vi "ReadFile.vi"(8 "error in (no error)":errorcluster, 11 "VXMCfg in":refnum<class "VXMCfg.lvclass">) -> (0 "error out":errorcluster, 3 "VXMCfg out":refnum<class "VXMCfg.lvclass">)   [LabVIEW 2018, in "VXMCfg.lvclass"]
uses:
  VXMCfg.lvclass
  VXMCfg.ctl
  sub-syst.n.ctl
  VXMCfg.lvclass/VXMCfg.ctl
panel:
  in  "VXM Properties":T1={"sub-syst1"={"Addr"="COM11", "Enable"=TRUE, "X scale eng./step"=0.00635, "Y scale eng./step"=0.00635, "Z scale eng./step"=0.0125, "T scale eng./step"=1.0, "X units"="mm", "Y units"="mm", "Z units"="deg", "T units"="", "X Jog"=1.0, "Y Jog"=1.0, "Z Jog"=1.0, "T Jog"=1.0, "X-1 Name"="", "Y-2 Name"="", "Z-3 Name"="", "T-4 Name"="", "VXM (1-4)"=3}, "sub-syst2"={"Addr"="", "Enable"=FALSE, "X scale eng./step"=0.00635, "Y scale eng./step"=0.00635, "Z scale eng./step"=0.0125, "T scale eng./step"=0.0125, "X units"="mm", "Y units"="mm", "Z units"="deg", "T units"="deg", "X Jog"=1.0, "Y Jog"=1.0, "Z Jog"=1.0, "T Jog"=1.0, "X-1 Name"="", "Y-2 Name"="", "Z-3 Name"="", "T-4 Name"="", "VXM (1-4)"=4}, "sub-syst3"={"Addr"="", "Enable"=FALSE, "X scale eng./step"=0.00635, "Y scale eng./step"=0.0125, "Z scale eng./step"=1.0, "T scale eng./step"=1.0, "X units"="mm", "Y units"="deg", "Z units"="", "T units"="", "X Jog"=1.0, "Y Jog"=1.0, "Z Jog"=1.0, "T Jog"=1.0, "X-1 Name"="", "Y-2 Name"="", "Z-3 Name"="", "T-4 Name"="", "VXM (1-4)"=2}}
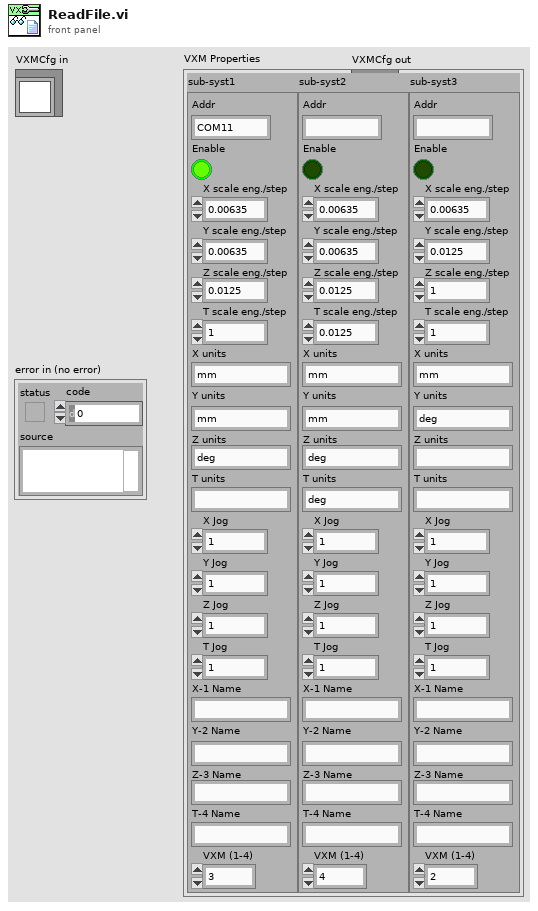
[diagram p1: front panel]
types:
  T1 = typedef "VXMCfg.ctl" = cluster{"sub-syst1":T2, "sub-syst2":T2, "sub-syst3":T2}
  T2 = typedef "sub-syst.n.ctl" = cluster{"Addr":string, "Enable":bool, "X scale eng./step":dbl, "Y scale eng./step":dbl, "Z scale eng./step":dbl, "T scale eng./step":dbl, "X units":string, "Y units":string, "Z units":string, "T units":string, "X Jog":dbl, "Y Jog":dbl, "Z Jog":dbl, "T Jog":dbl, "X-1 Name":string, "Y-2 Name":string, "Z-3 Name":string, "T-4 Name":string, "VXM (1-4)":i32}
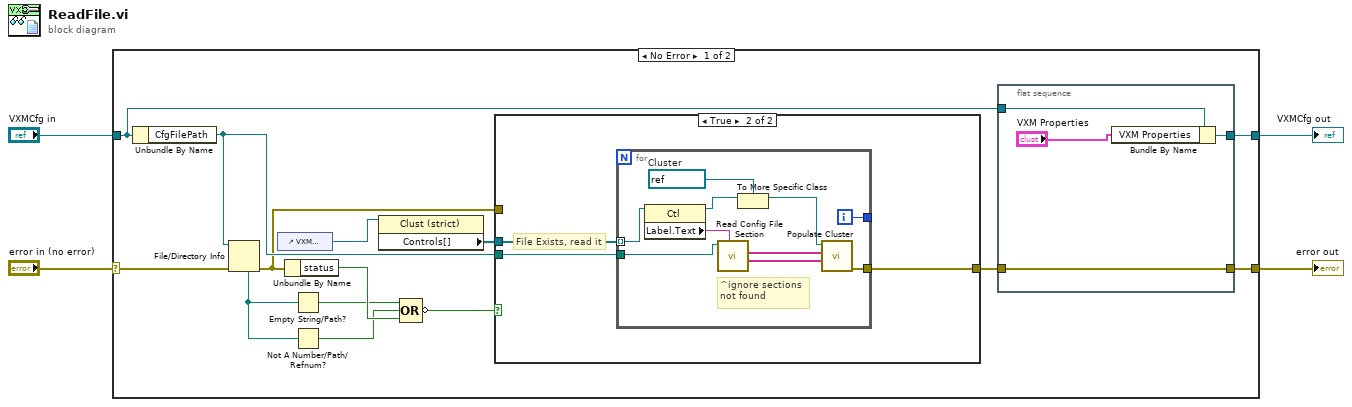
[diagram p0: block diagram]
diagram:
  n1 = case shown="No Error" "error in (no error)" {
    selector: "error in (no error)" -> [w10 w38]
    tunnel: [w9 w38] -> w2
    tunnel: [w11 w37] -> w1
    tunnel: "VXMCfg in" -> [w7 w37]
    frame No Error {
      n2 = Unbundle By Name(w7) -> ("CfgFilePath"=w6:path)
      n3 = File/Directory Info(path=w6, error in=w10) -> (error out=w5:errorcluster, resolved path=w12:path)  [unwired: 5 out]
      n4 = control-ref of="VXM Properties"() -> (w8:refnum<vi>)
      n5 = Unbundle By Name(w5) -> ("status"=w15:bool)
      n6 = Empty String/Path?(string/path=w12) -> (empty?=w13:bool)
      n7 = Not A Number/Path/Refnum?(number/path/refnum=w12) -> (NaN/Path/Refnum?=w14:bool)
      n8 = property class="Clust (strict)"(reference=w8) -> ("Controls[]"=w16:refnum<vi>[])  [unwired: 1 in, 2 out]
      n9 = Compound Arithmetic op=OR(w13, w14, w15) -> (invert w17:bool)
      n10 = case shown="True" w17 {
        tunnel: w6 -> [_ w26]
        tunnel: w16 -> [_ w25]
        tunnel: [w23 w24] -> w18
        tunnel: w5 -> [w23 _]
        frame False {
          # "no file, don't read"
        }
        frame True {
          # "File Exists, read it"
          n11 = for {
            tunnel: w25 -> [w36] mode=indexing
            tunnel: w26 -> [w34]
            tunnel: [w31] -> w24
            tunnel: [w27] -> _
            i -> [w27]
            w30 = refnum<vi> refnum  # Cluster
            # "^ignore sections\nnot found"
            n12 = property class="Ctl"(reference=w36) -> (reference out=w29:refnum<vi>, "Label.Text"=w35:string)  [unwired: 1 in, 1 out]
            n13 = call "Read Config File Section.vi"("Section"=w35, "appended path"=w34) -> ("Values"=w32:string[], "Keys"=w33:string[])  [unwired: 7 in, 1 out]
            n14 = To More Specific Class(target class=w30, reference=w29) -> (specific class reference=w28:refnum<vi>)  [unwired: 1 in, 1 out]
            n15 = call "Populate Cluster.vi"("Values"=w32, "Keys"=w33, "Clust Refnum"=w28) -> ("error out"=w31:errorcluster)  [unwired: 7 in, 1 out]
          }
        }
      }
      n16 = flat-sequence {
        tunnel: w7 -> [w22]
        tunnel: [w21] -> w11
        tunnel: [w20] -> w9
        tunnel: w18 -> [w20]
        frame #0 {
          n17 = Bundle By Name(cluster=w22, "VXM Properties"="VXM Properties") -> (w21:refnum<class "VXMCfg.lvclass">)
        }
      }
    }
    frame Error {
    }
  }
  "error out" <- w2
  "VXMCfg out" <- w1
